vi "combined arm safety.vi"(7 "Input":dbl) -> (8 "Safe Output":dbl, 13 "Safety":cluster{"Arm Safety":bool, "Arm Limit":bool}={"Arm Safety"=TRUE, "Arm Limit"=FALSE})   [LabVIEW 2013]
panel:
  in  "Min Rate":dbl format="%#_13g"
  in  "Max Rate":dbl=50.0 format="%#_13g"
  in  "Forward Limit":dbl format="%#_13g"
  in  "Reverse Limit":dbl format="%#_13g"
  in  "Cutoff Rate":dbl=0.8 format="%#_13g"
  # "Things needing Tuning"
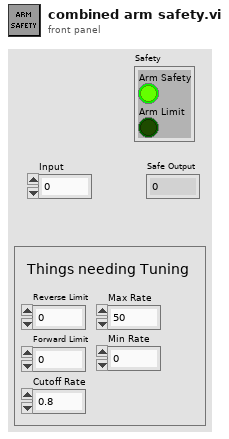
[diagram p1: front panel]
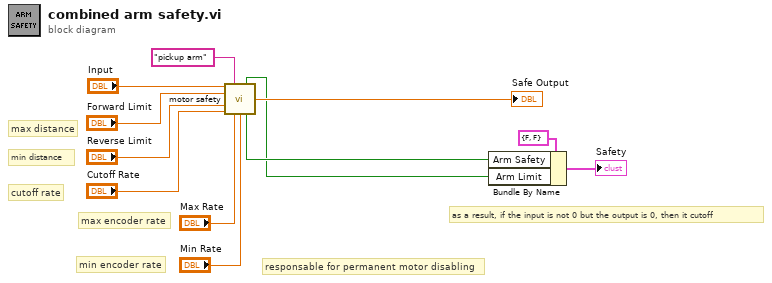
[diagram p0: block diagram]
diagram:
  # "as a result, if the input is not 0 but the output is 0, then it cutoff"
  # "responsable for permanent motor disabling"
  # "min encoder rate"
  # "max encoder rate"
  # "cutoff rate"
  # "min distance"
  # "max distance"
  n1 = call "motor safety.vi"("Desired Rate"="Input", "Encoder Refnum"="pickup arm", "Forward Limit"="Forward Limit", "Reverse Limit"="Reverse Limit", "Cutoff Rate"="Cutoff Rate", "Max Rate"="Max Rate", "Min Rate"="Min Rate") -> ("Limit"=w1:bool, "Rate Output"=→"Safe Output":dbl, "Cutoff Tripped"=w2:bool)  [unwired: 6 in]
  n2 = Bundle By Name(cluster=cluster{"Arm Safety":bool, "Arm Limit":bool} {"Arm Safety"=FALSE, "Arm Limit"=FALSE} ("Input"), "Arm Safety"=w2, "Arm Limit"=w1) -> (→"Safety":cluster{"Arm Safety":bool, "Arm Limit":bool})
